vi "Teleop.vi"(10 "Match Info":T1={"Autonomous Elapsed Seconds"=0.0, "TeleOp Elapsed Seconds"=0.0, "Disabled Elapsed Seconds"=0.0, "Visited Autonomous"=FALSE, "Visited TeleOp"=FALSE, "Visited Disabled"=FALSE, "Autonomous Settings"={"Autonomous Style"=enum."Independent", "VI Refnum"=refnum}}, 11 "Call Context":T2) -> ()   [LabVIEW 2017]
doc: "This VI is called for each TeleOp packet received from the DS where the robot is not disabled. It is often used to read from the joysticks and update I/O or to update setpoints for timed control loops. It should complete and return within 20 milliseconds or it may miss DS packets."
uses:
  <vilib>/Rock Robotics/WPI/DriverStation/WPI_DriverStationDerivedRobotMode.ctl
  <vilib>/Rock Robotics/WPI/DriverStation/WPI_DriverStationMatch Info.ctl
  <vilib>/Rock Robotics/WPI/Utilities/WPI_GetSetVariantRefNum.vi
  Robot Global Data.vi
  <vilib>/Rock Robotics/Network Tables/NT Write Boolean Array.vi
  <vilib>/Rock Robotics/Network Tables/NT Write Numeric Array.vi
  <vilib>/Rock Robotics/Network Tables/NT Write Boolean.vi
panel:
  out "Compressor Running":bool
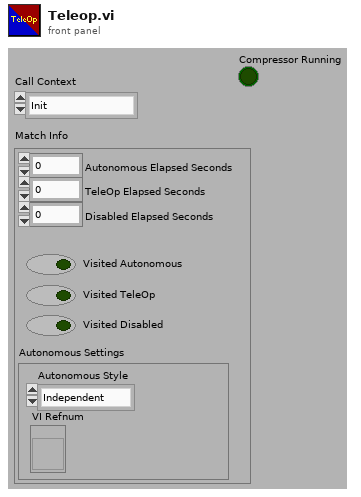
[diagram p1: front panel]
types:
  T1 = typedef "WPI_DriverStationMatch Info.ctl" = cluster{"Autonomous Elapsed Seconds":dbl, "TeleOp Elapsed Seconds":dbl, "Disabled Elapsed Seconds":dbl, "Visited Autonomous":bool, "Visited TeleOp":bool, "Visited Disabled":bool, "Autonomous Settings":cluster{"Autonomous Style":enum16{"Iterative", "Independent"}, "VI Refnum":refnum<vi>}}
  T2 = typedef "WPI_DriverStationDerivedRobotMode.ctl" = enum16{"Init", "Execute", "Stop"}
  T3 = typedef "WPI_JoystickDevRef.ctl" = cluster{"Device":T4}
  T4 = typedef "WPI_JoystickDeviceEnum.ctl" = enum16{"USB 0", "USB 1", "USB 2", "USB 3", "USB 4", "USB 5"}
  T5 = typedef "WPI_CompressorDevRef.ctl" = cluster{"DevStatus":errorcluster, "Pneumatics Control Module":u8}
  T6 = typedef "WPI_MotorControlDeviceRef.ctl" = cluster{"DeviceStatus":errorcluster, "Type":T7, "PWM":cluster{"PWM Channel":T8, "DeadBand":T9}, "CAN":cluster{"Device Number":u8, "SetOutput VI Ref":variant, "GetOutput VI Ref":variant, "Enable VI Ref":variant, "Disable VI Ref":variant, "Data":variant}, "Invert":bool, "DIO PWM":cluster{"PWM \"Enable\" Channel":T8, "DIOChannel":T10, "PWM Rate":dbl}}
  T7 = typedef "WPI_MotorControlType.ctl" = enum16{"PWM", "CAN", "DIO PWM"}
  T8 = typedef "FPGA_DIOPWMChannel.ctl" = enum8{"PWM 0", "PWM 1", "PWM 2", "PWM 3", "PWM 4", "PWM 5", "PWM 6", "PWM 7", "PWM 8", "PWM 9", "PWM MXP 0", "PWM MXP 1", "PWM MXP 2", "PWM MXP 3", "PWM MXP 4", "PWM MXP 5", "PWM MXP 6", "PWM MXP 7", "PWM MXP 8", "PWM MXP 9", "Invalid"}
  T9 = typedef "WPI_PWMDeadband.ctl" = cluster{"Name":string, "maxPositivePwm":i32, "minPositivePwm":i32, "centerPwm":i32, "maxNegativePwm":i32, "minNegativePwm":i32, "angularRange":u16}
  T10 = typedef "FPGA_DIOChannel.ctl" = enum8{"DIO 0", "DIO 1", "DIO 2", "DIO 3", "DIO 4", "DIO 5", "DIO 6", "DIO 7", "DIO 8", "DIO 9", "DIO MXP 0", "DIO MXP 1", "DIO MXP 2", "DIO MXP 3", "DIO MXP 4", "DIO MXP 5", "DIO MXP 6", "DIO MXP 7", "DIO MXP 8", "DIO MXP 9", "DIO MXP 10", "DIO MXP 11", "DIO MXP 12", "DIO MXP 13", "DIO MXP 14", "DIO MXP 15", "SPI Port CS1", "SPI Port CS2", "SPI Port CS3", "SPI Port MISO", "SPI Port MOSI", "Invalid"}
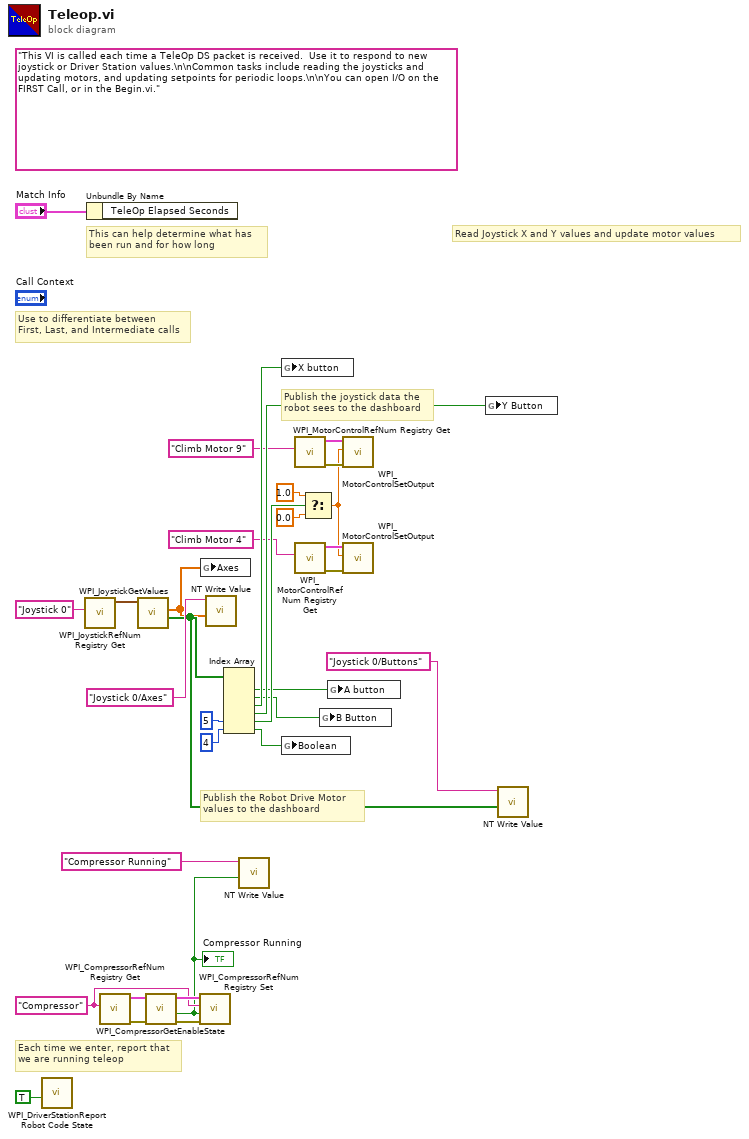
[diagram p0: block diagram]
diagram:
  w7 = "Compressor" ("refnum name")
  (unwired) "This VI is called each time a TeleOp DS packet is received.  Use it to respond to new joystick or Driver Station values.\n\nCommon tasks include reading the joysticks and updating motors, and updating setpoints for periodic loops.\n\nYou can open I/O on the FIRST Call, or in the Begin.vi."
  # "Publish the Robot Drive Motor\nvalues to the dashboard"
  # "Publish the joystick data the\nrobot sees to the dashboard"
  # "Each time we enter, report that\nwe are running teleop"
  # "Use to differentiate between\nFirst, Last, and Intermediate calls"
  # "This can help determine what has\nbeen run and for how long"
  # "Read Joystick X and Y values and update motor values"
  n1 = call <vilib>:"WPI_DriverStationReport Robot Code State.vi"("TeleOp"=TRUE ("Autonomous")) -> ()  [unwired: 10 in, 1 out]
  n2 = call <vilib>:"WPI_JoystickRefNum Registry Get.vi"("refnum name"="Joystick 0") -> ("JoystickDevRef"=w30:T3)  [unwired: 1 in, 9 out]
  n3 = Unbundle By Name("Match Info") -> ()  [unwired: 1 out]
  n4 = call <vilib>:"WPI_CompressorRefNum Registry Get.vi"("refnum name"=w7) -> ("error out"=w11:errorcluster, "CompressorDevRef"=w10:T5)  [unwired: 9 in]
  n5 = call <vilib>:"WPI_JoystickGetValues.vi"("JoystickDevRef"=w30) -> ("Buttons"=w26:bool[], "Axes"=w25:dbl[])  [unwired: 6 in, 3 out]
  n6 = call <vilib>:"WPI_CompressorGetEnableState.vi"("error in (no error)"=w11, "CompressorDevRef"=w10) -> ("error out"=w9:errorcluster, "Compressor Running"=w6:bool, "CompressorDevRef"=w8:T5)  [unwired: 6 in, 1 out]
  "Compressor Running" <- w6
  n7 = call <vilib>:"WPI_CompressorRefNum Registry Set.vi"("error in (no error)"=w9, "Test Mode Only"=w6, "refnum name"=w7, "CompressorDevRef"=w8) -> ()  [unwired: 6 in, 2 out]
  n8 = global write "Robot Global Data.vi" "Axes"(w25) -> ()
  n9 = call-poly <vilib>:"NT Write Value.vi"("Numeric Array"=w25, "Name"="Joystick 0/Axes") -> ()  [unwired: 9 in, 1 out]
  n10 = Index Array(array=w26, index #5=5 ("index"), index #6=4 ("index")) -> (element #1=w2:bool, element #2=w1:bool, element #3=w24:bool, element #4=w23:bool, element #5=w21:bool, element #6=w3:bool)  [unwired: 4 in]
  n11 = call-poly <vilib>:"NT Write Value.vi"("Boolean"=w6, "Name"="Compressor Running") -> ()  [unwired: 9 in, 1 out]
  n12 = global write "Robot Global Data.vi" "X button"(w24) -> ()
  n13 = global write "Robot Global Data.vi" "Boolean"(w3) -> ()
  n14 = call <vilib>:"WPI_MotorControlRefNum Registry Get.vi"("refnum name"="Climb Motor 9") -> ("error out"=w14:errorcluster, "MotorControlDevRef"=w13:T6)  [unwired: 9 in]
  n15 = call <vilib>:"WPI_MotorControlRefNum Registry Get.vi"("refnum name"="Climb Motor 4") -> ("error out"=w18:errorcluster, "MotorControlDevRef"=w17:T6)  [unwired: 9 in]
  n16 = Select(t=1.0, s=w21, f=0.0) -> (s? t:f=w12:dbl)
  n17 = global write "Robot Global Data.vi" "B Button"(w1) -> ()
  n18 = global write "Robot Global Data.vi" "A button"(w2) -> ()
  n19 = call <vilib>:"WPI_MotorControlSetOutput.vi"("error in (no error)"=w14, "Output"=w12, "MotorControlDevRef"=w13) -> ()  [unwired: 6 in, 3 out]
  n20 = call <vilib>:"WPI_MotorControlSetOutput.vi"("error in (no error)"=w18, "Output"=w12, "MotorControlDevRef"=w17) -> ()  [unwired: 6 in, 3 out]
  n21 = global write "Robot Global Data.vi" "Y Button"(w23) -> ()
  n22 = call-poly <vilib>:"NT Write Value.vi"("Boolean Array"=w26, "Name"="Joystick 0/Buttons") -> ()  [unwired: 9 in, 1 out]
